vi "Specify Path Enum.vi"(9 "Icon Editor Invoker Type":T2) -> (1 "Path":T1)   [LabVIEW 2021]
uses:
  <resource>/plugins/Icon Editor Invoker Type.ctl
  <vilib>/LabVIEW Icon API/lv_icon/Controls/Pathes.ctl
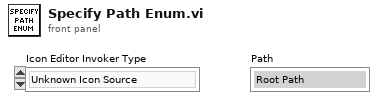
[diagram p1: front panel]
types:
  T1 = typedef "Pathes.ctl" = enum16{"Root Path", "Icon Templates", "Icon Templates VI", "Icon Templates Lib", "Glyphs"}
  T2 = typedef "Icon Editor Invoker Type.ctl" = enum32{"Unknown Icon Source", "VI Icon", "Library Icon (any library type)", "Palette icon", "Icon from App Method"}
  T3 = enum32{"Unknown Icon Source", "VI Icon", "Library Icon (any library type)", "Palette icon", "Icon from App Method"}
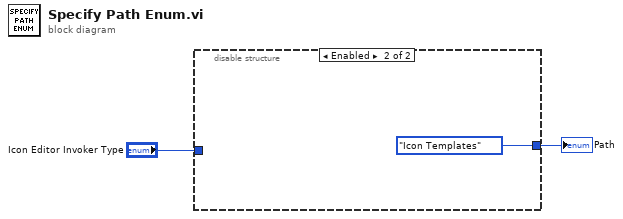
[diagram p0: block diagram]
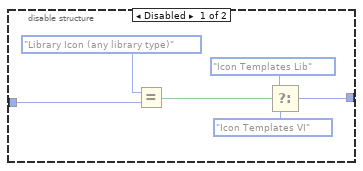
[diagram p2: hidden frame]
diagram:
  n1 = disable-structure shown="Enabled" {
    disable-tunnel: "Icon Editor Invoker Type" -> [w8 _]
    disable-tunnel: [w6 Pathes."Icon Templates" ("Path")] -> w1
    frame Disabled {
      n2 = Equal?(x=T3."Library Icon (any library type)", y=w8) -> (x = y?=w5:bool)
      n3 = Select(t=Pathes."Icon Templates Lib" ("Path"), s=w5, f=Pathes."Icon Templates VI" ("Path")) -> (s? t:f=w6:T1)
    }
    frame Enabled {
    }
  }
  "Path" <- w1
